vi "main.vi"() -> ()   [LabVIEW 2010]
uses:
  subVIs/XML_repo_library.lvlib
panel:
  out "MainLoop_state":T1(ring)
  in  "Tab Control":T2(tab)
  in  "Measure with":dbl(ring) items=["0. Demo Nanopositioner Stage 1.0", "0. Demo Avalanche Photodiode 1.0"]
  in  "Scan with":dbl(ring) items=["0. Demo Nanopositioner Stage 1.0", "0. Demo Avalanche Photodiode 1.0"]
  in  "stop":bool
  in  "start":bool
  in  "quit":bool
  out "Intensity Graph":dbl[][](graph)
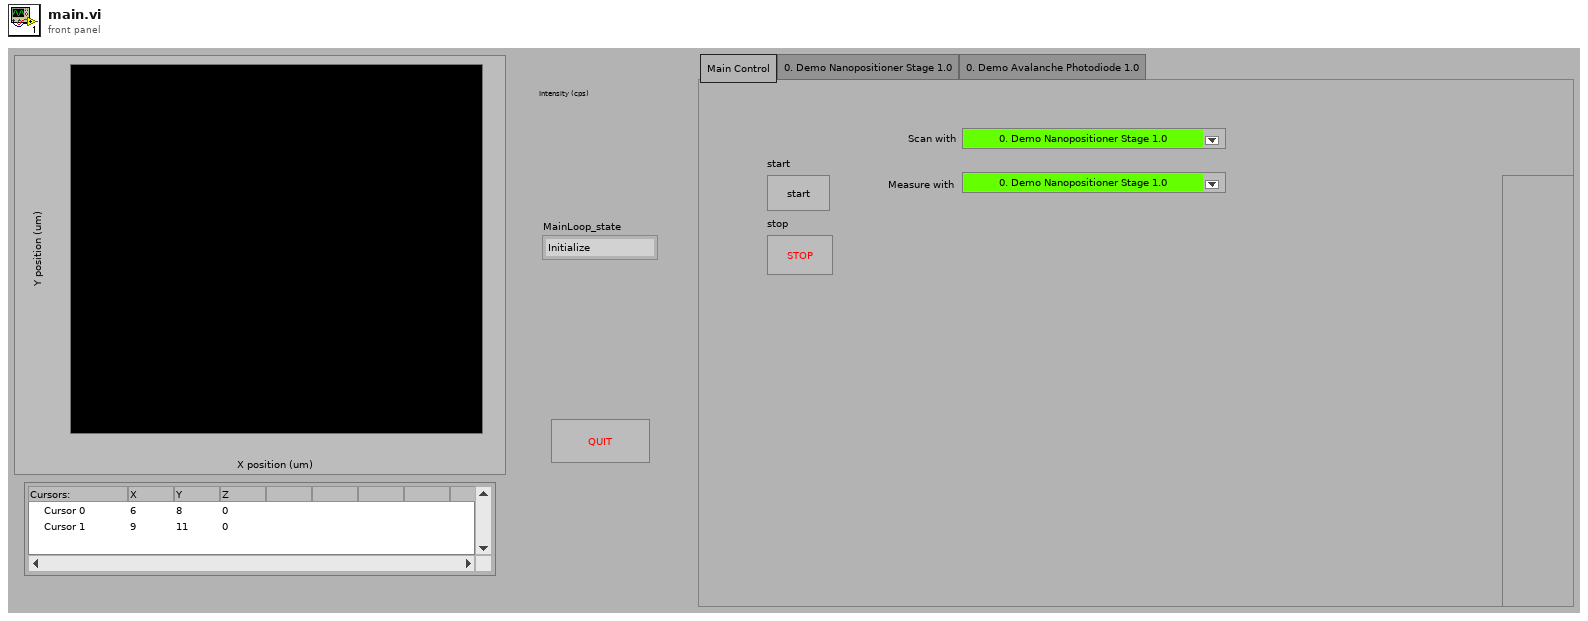
[diagram p1: front panel]
types:
  T1 = enum16{"Initialize", "Setup Elements", "IDLE", "Acquire", "Save to file", "Deinitialize", "Shutdown", ""}
  T2 = enum32{"Page 1", "Page 6", "Page 2", "Page 3", "Page 4", "Page 5", "Page 7", "Page 8"}
  T3 = cluster{"Name":string, "Setup_element_type":enum16{"positioner", "acquisition", "synchronized"}, "VIpath":path, "Return type":string, "Stage info":cluster{"Value":string, i32, "node text":string}[], "Number":u32, "Setup_element_direction":enum16{"output", "input", "io"}}[]
  T4 = cluster{"Name":string, "Setup_element_type":enum16{"positioner", "acquisition", "synchronized"}, "VIpath":path, "Return type":string, "Stage info":cluster{"Value":string, i32, "node text":string}[], "Number":u32, "Setup_element_direction":enum16{"output", "input", "io"}}
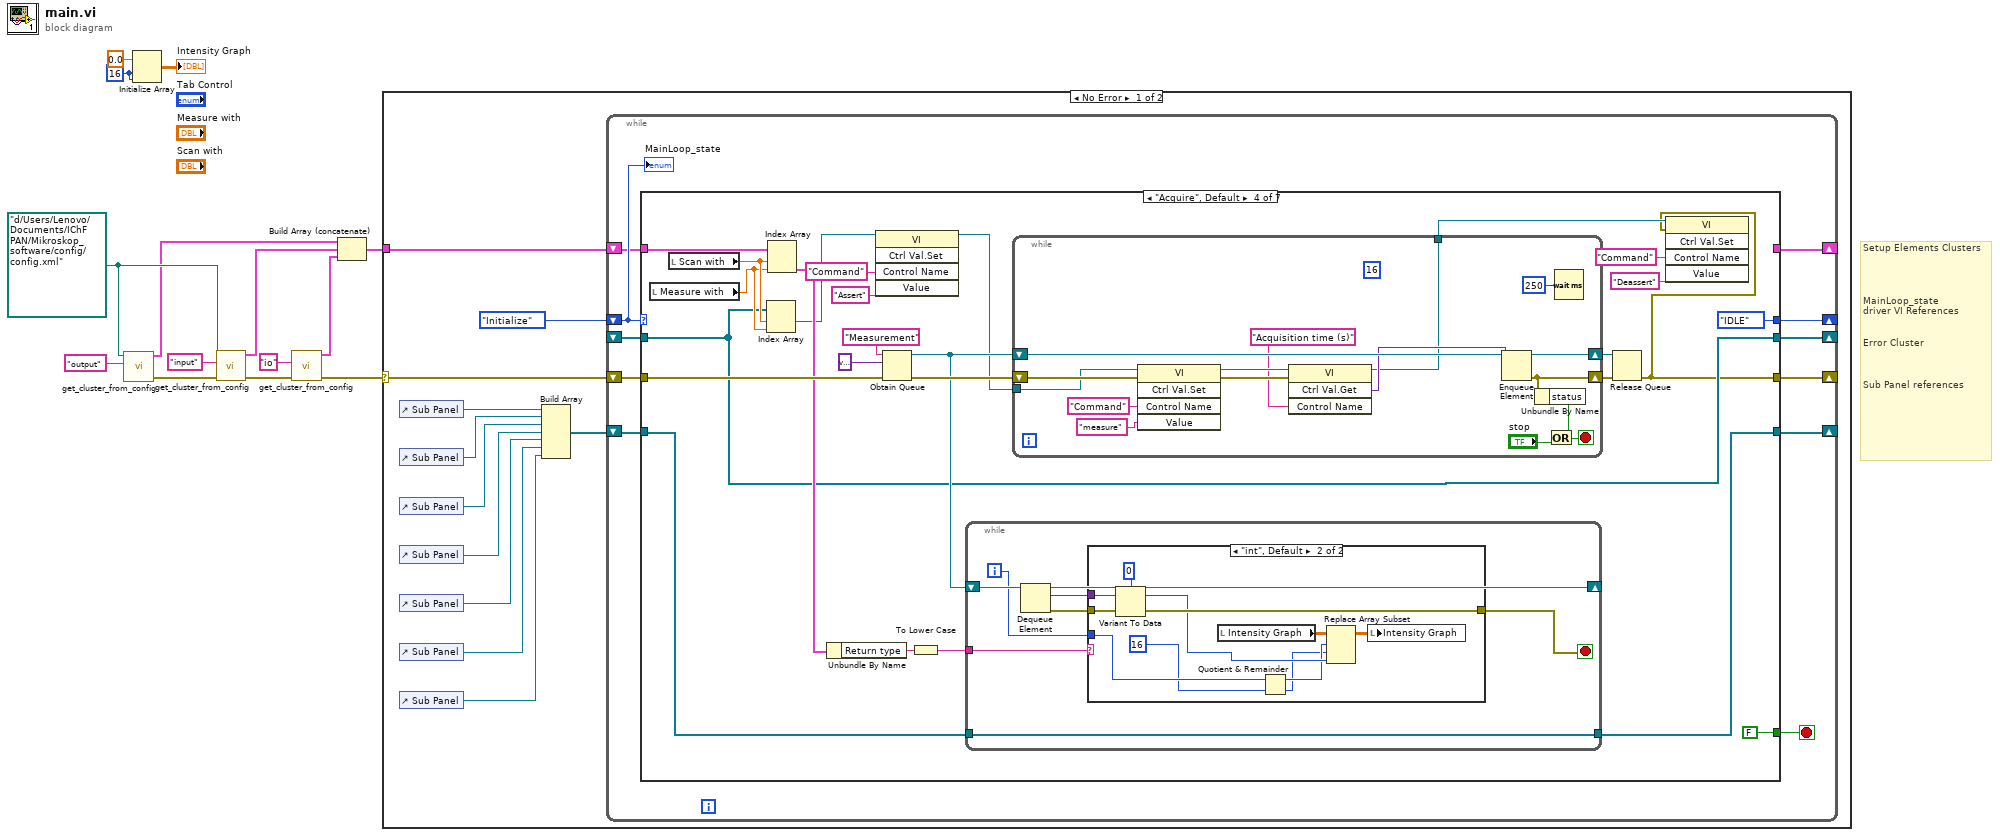
[diagram p0: block diagram]
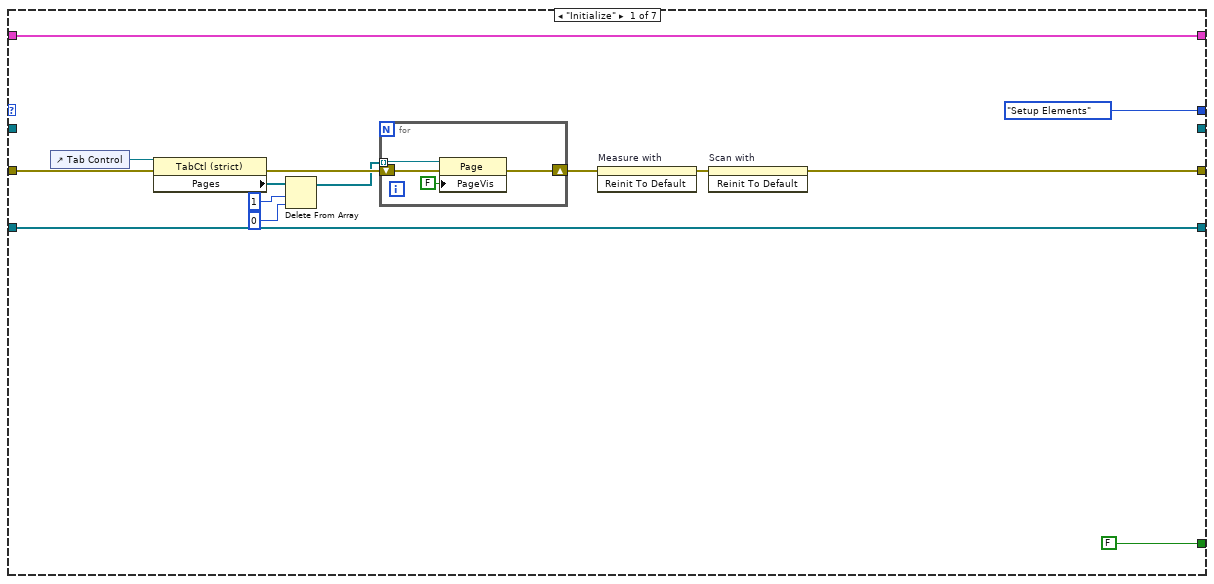
[diagram p2: hidden frame]
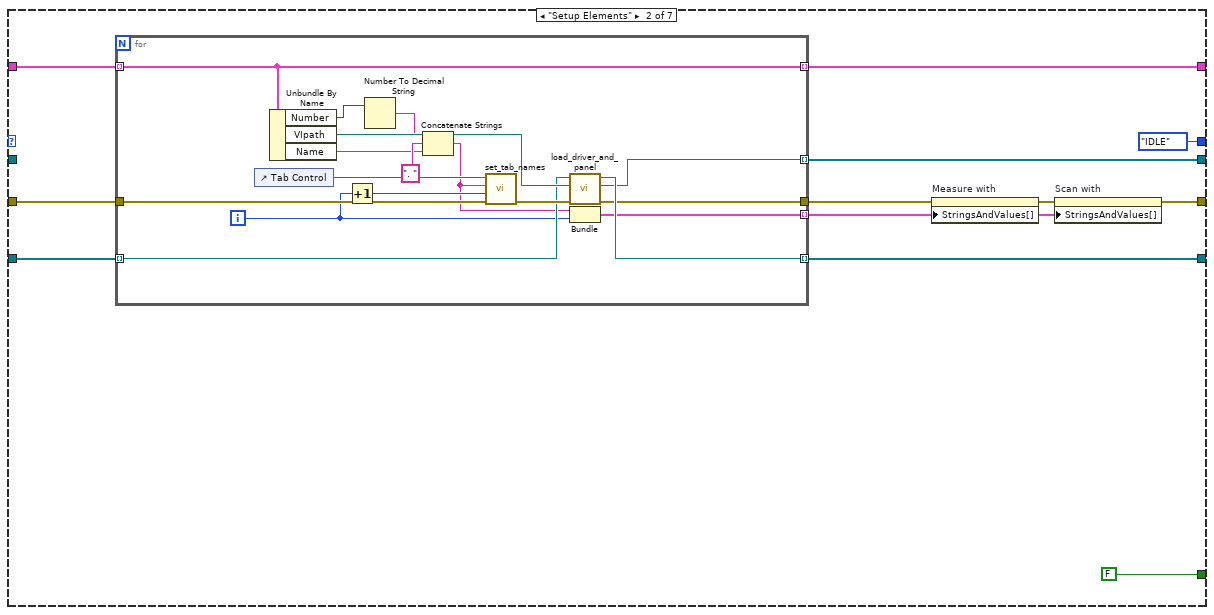
[diagram p3: hidden frame]
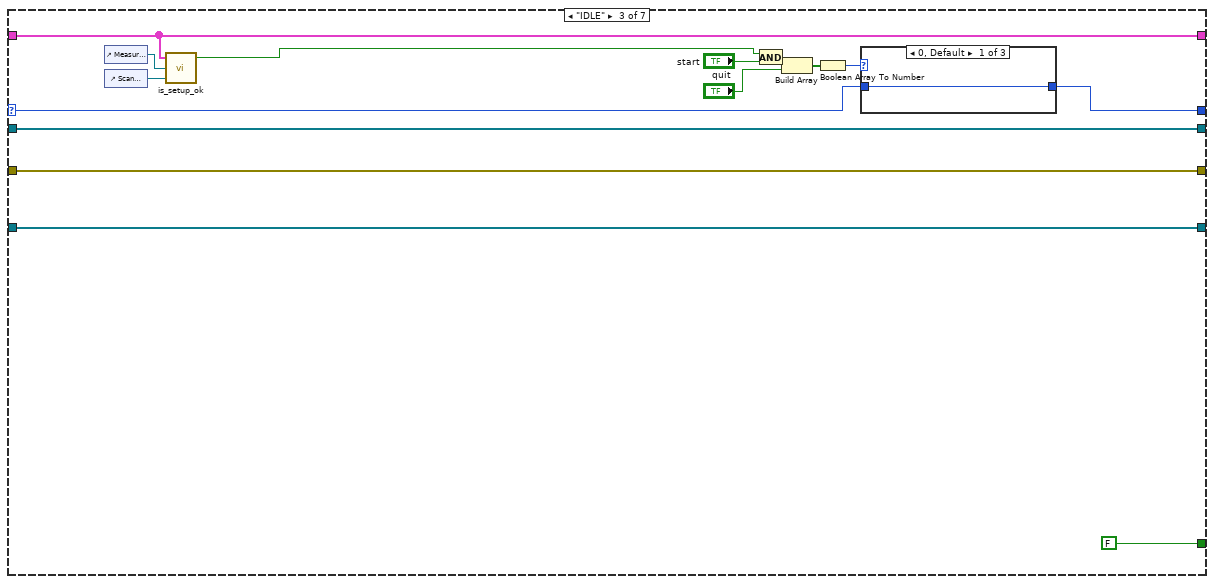
[diagram p4: hidden frame]
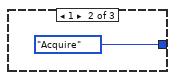
[diagram p5: hidden frame]
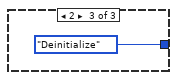
[diagram p6: hidden frame]
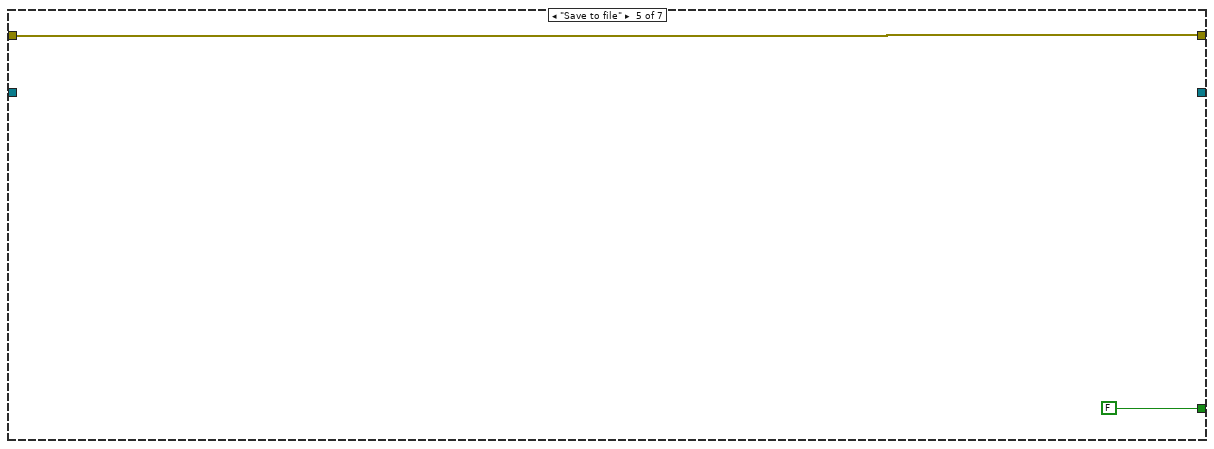
[diagram p8: hidden frame]
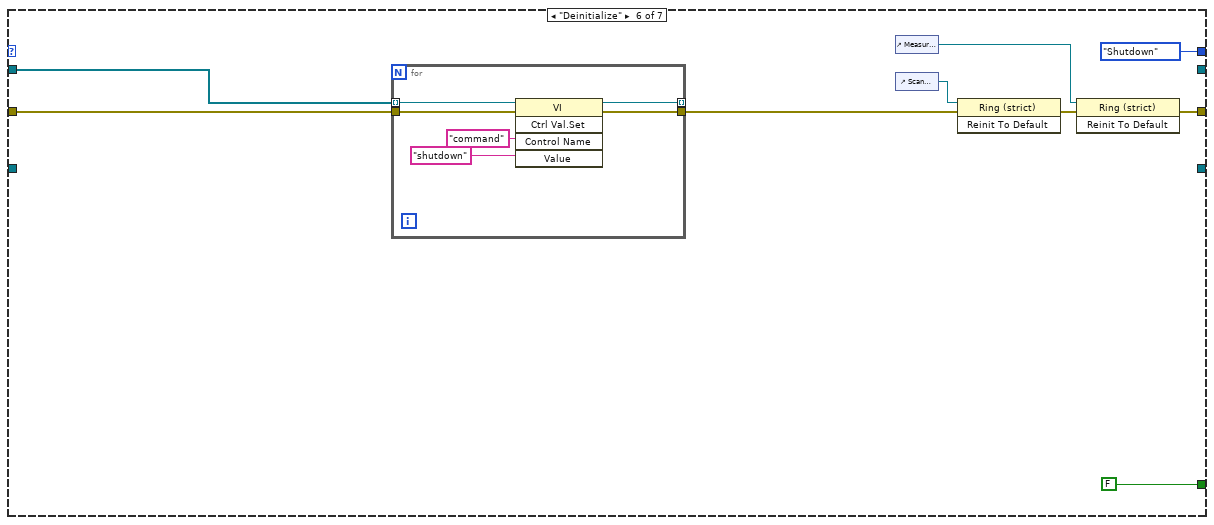
[diagram p9: hidden frame]
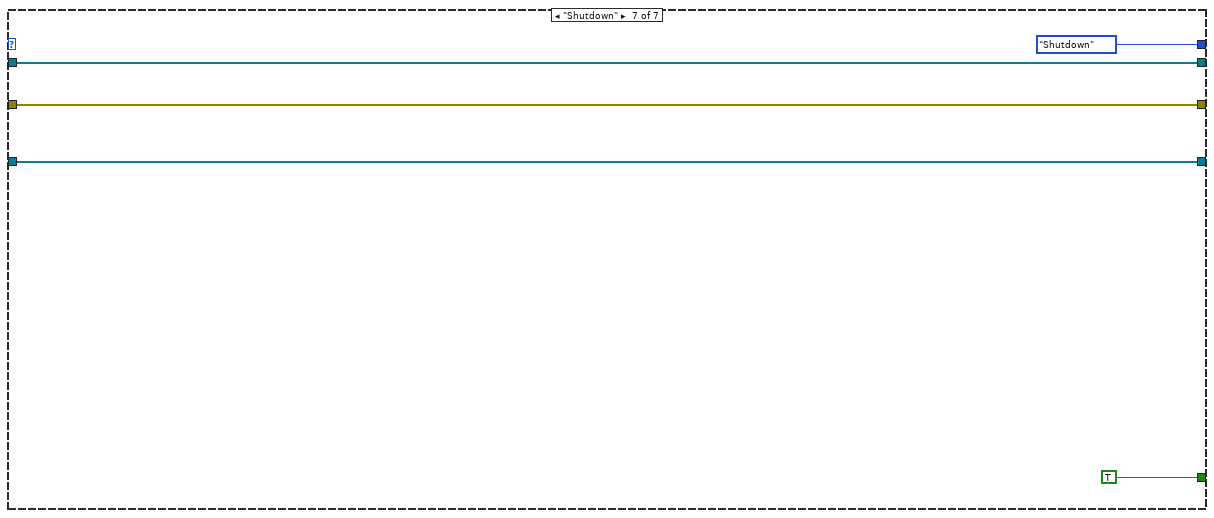
[diagram p10: hidden frame]
diagram:
  w1 = 16 ("dimension size")
  w12 = path "d:/Users/Lenovo/Documents/IChF PAN/Mikroskop_software/config/config.xml" ("path to XML document")
  # "Setup Elements Clusters\n\n\n\n\nMainLoop_state\ndriver VI References\n\n\nError Cluster\n\n\n\nSub Panel references"
  n1 = call "get_cluster_from_config.vi"("microscope tag type"="output" ("XPath expression"), "path to config file"=w12) -> ("error out"=w13:errorcluster, "Array"=w8:T3)  [unwired: 4 in]
  n2 = Initialize Array(0.0 ("element"), w1, w1) -> (→"Intensity Graph":dbl[][])
  n3 = call "get_cluster_from_config.vi"("error in (no error)"=w13, "microscope tag type"="input", "path to config file"=w12) -> ("error out"=w10:errorcluster, "Array"=w6:T3)  [unwired: 3 in]
  n4 = call "get_cluster_from_config.vi"("error in (no error)"=w10, "microscope tag type"="io") -> ("error out"=w4:errorcluster, "Array"=w5:T3)  [unwired: 4 in]
  n5 = Build Array (concatenate)(w8, w6, w5) -> (w7:T3)
  n6 = case shown="No Error" w4 {
    selector: w4 -> [w24 _]
    tunnel: w7 -> [w25 _]
    frame No Error {
      n7 = control-ref of="Sub Panel"() -> (w16:refnum<vi>)
      n8 = control-ref of="Sub Panel"() -> (w17:refnum<vi>)
      n9 = control-ref of="Sub Panel"() -> (w18:refnum<vi>)
      n10 = control-ref of="Sub Panel"() -> (w19:refnum<vi>)
      n11 = control-ref of="Sub Panel"() -> (w20:refnum<vi>)
      n12 = control-ref of="Sub Panel"() -> (w21:refnum<vi>)
      n13 = control-ref of="Sub Panel"() -> (w22:refnum<vi>)
      n14 = Build Array(w16, w17, w18, w19, w20, w21, w22) -> (w15:refnum<vi>[])
      n15 = while {
        shift-right: [w36] -> _
        shift-left: T1."Initialize" ("MainLoop_state") -> [w35]
        shift-right: [w33] -> _
        shift-left: w24 -> [w34]
        shift-right: [w30] -> _
        shift-left: w15 -> [w31]
        shift-right: [w29] -> _
        shift-left: w25 -> [w32]
        shift-right: [w27] -> _
        shift-left: _ -> [w26]
        stop <- w28 stop-if-true
        n16 = case shown="\"Acquire\", Default" w35 {
          selector: w35 -> [_ _ w89 _ _ _ _]
          tunnel: [T1."Setup Elements" ("MainLoop_state") T1."IDLE" ("MainLoop_state") w93 T1."IDLE" ("MainLoop_state") _ T1."Shutdown" ("MainLoop_state") T1."Shutdown" ("MainLoop_state")] -> w36
          tunnel: w34 -> [w44 w66 w90 w114 w165 w168 w182]
          tunnel: [w37 w55 w90 w102 w165 w171 w182] -> w33
          tunnel: w32 -> [w41 w62 w88 w116 _ _ _]
          tunnel: w31 -> [w42 w64 w98 w122 _ _ w181]
          tunnel: [w42 w63 w98 w123 _ _ w181] -> w30
          tunnel: [w41 w59 w88 _ _ _ _] -> w29
          tunnel: [FALSE FALSE FALSE FALSE FALSE FALSE TRUE] -> w28
          tunnel: [_ w60 w91 w110 _ _ w183] -> w27
          tunnel: w26 -> [_ _ w91 w110 _ w166 w183]
          frame "Initialize" {
            n17 = control-ref of="Tab Control"() -> (w50:refnum<vi>)
            n18 = property class="TabCtl (strict)"(reference=w50, error in=w44) -> (error out=w49:errorcluster, "Pages"=w48:refnum<vi>[])  [unwired: 1 out]
            n19 = Delete From Array(array=w48, length=1, index=0) -> (array with subset deleted=w47:refnum<vi>[])  [unwired: 1 out]
            n20 = for {
              tunnel: w47 -> [w53] mode=indexing
              shift-right: [w51] -> w38
              shift-left: w49 -> [w52]
              n21 = property class="Page"(reference=w53, error in=w52, "PageVis"=FALSE ("Page Visible")) -> (error out=w51:errorcluster)  [unwired: 1 out]
            }
            n22 = invoke on="Measure with" class="Ring (strict)" method="Reinit To Default"(error in=w38) -> (error out=w39:errorcluster)  [unwired: 2 in, 2 out]
            n23 = invoke on="Scan with" class="Ring (strict)" method="Reinit To Default"(error in=w39) -> (error out=w37:errorcluster)  [unwired: 2 in, 2 out]
          }
          frame "Setup Elements" {
            n24 = for {
              tunnel: w66 -> [w83]
              tunnel: [w67] -> w58
              tunnel: w62 -> [w72] mode=indexing
              tunnel: w64 -> [w77] mode=indexing
              tunnel: [w78] -> w63 mode=indexing
              tunnel: [w76] -> w60 mode=indexing
              tunnel: [w72] -> w59 mode=indexing
              tunnel: [w71] -> w56 mode=indexing
              i -> [w69]
              n25 = control-ref of="Tab Control"() -> (w82:refnum<vi>)
              n26 = Unbundle By Name(w72) -> ("Number"=w68:u32, "VIpath"=w79:path, "Name"=w73:string)
              n27 = Increment(x=w69) -> (x+1=w80:i32)
              n28 = Number To Decimal String(number=w68) -> (decimal integer string=w74:string)  [unwired: 1 in]
              n29 = Concatenate Strings(w74, ". " ("string"), w73) -> (w70:string)
              n30 = call "set_tab_names.vi"("error out 2"=w83, "index"=w80, "Name"=w70, "Tab Control"=w82) -> ("error out"=w81:errorcluster)  [unwired: 3 in]
              n31 = call "load_driver_and_panel.vi"("error in (no error)"=w81, "VIpath"=w79, "Sub Panel in"=w77) -> ("error out"=w67:errorcluster, "driver VI Refnum"=w76:refnum<vi>, "Sub Panel out"=w78:refnum<vi>)  [unwired: 2 in]
              n32 = Bundle(w70, w69) -> (w71:cluster{string, i32})  [unwired: 1 in]
            }
            n33 = property on="Measure with" class="Ring (strict)"(error in=w58, "StringsAndValues[]"=w56) -> (error out=w57:errorcluster)  [unwired: 1 in, 1 out]
            n34 = property on="Scan with" class="Ring (strict)"(error in=w57, "StringsAndValues[]"=w56) -> (error out=w55:errorcluster)  [unwired: 1 in, 1 out]
          }
          frame "IDLE" {
            n35 = control-ref of="Measure with"() -> (w86:refnum<vi>)
            n36 = control-ref of="Scan with"() -> (w85:refnum<vi>)
            n37 = call "is_setup_ok.vi"("Scan with"=w85, "Measure with"=w86, "Array"=w88) -> ("All OK"=w84:bool)  [unwired: 2 out]
            n38 = And(x=w84, y="start") -> (x .and. y?=w87:bool)
            n39 = Build Array(w87, "quit") -> (w95:bool[])
            n40 = Boolean Array To Number(Boolean array=w95) -> (number=w94:u32)
            n41 = case shown="0, Default" w94 {
              tunnel: [w99 T1."Acquire" ("MainLoop_state") T1."Deinitialize" ("MainLoop_state")] -> w93
              tunnel: w89 -> [w99 _ _]
              frame 0, Default {
              }
              frame 1 {
              }
              frame 2 {
              }
            }
          }
          frame "Acquire", Default {
            n42 = local read "Measure with"() -> (w111:dbl)
            n43 = local read "Scan with"() -> (w112:dbl)
            n44 = Index Array(array=w110, index #1=w112, index #2=w111) -> (element #1=w109:refnum<vi>)  [unwired: 1 out]
            n45 = Index Array(array=w116, index #1=w112, index #2=w111) -> (element #2=w113:T4)  [unwired: 1 out]
            n46 = Unbundle By Name(w113) -> ("Return type"=w115:string)
            n47 = invoke class="VI" method="Ctrl Val.Set"(reference=w109, "Control Name"="Command", "Value"="Assert" ("Control Name")) -> (reference out=w106:refnum<vi>)  [unwired: 2 in, 4 out]
            n48 = Obtain Queue(name (unnamed)="Measurement", element data type=variant ("variant"), error in (no error)=w114) -> (queue out=w126:refnum<queue>, error out=w127:errorcluster)  [unwired: 2 in, 1 out]
            n49 = To Lower Case(string=w115) -> (all lower case string=w117:string)
            n50 = while {
              shift-right: [w134] -> _
              shift-left: w126 -> [w135]
              tunnel: [w133] -> w123
              tunnel: w122 -> [w133]
              tunnel: w117 -> [w132]
              i -> [w128]
              stop <- w129 stop-if-true
              n51 = Dequeue Element(queue=w135) -> (queue out=w134:refnum<queue>, element=w131:variant, error out=w130:errorcluster)  [unwired: 2 in, 1 out]
              n52 = case shown="\"int\", Default" w132 {
                tunnel: w131 -> [_ w146]
                tunnel: w130 -> [w136 w145]
                tunnel: [w136 w144] -> w129
                tunnel: w128 -> [_ w140]
                frame "False" {
                }
                frame "int", Default {
                  n53 = Variant To Data(error in=w145, Variant=w146, type=0) -> (error out=w144:errorcluster, data=w141:i32)
                  n54 = local read "Intensity Graph"() -> (w142:dbl[][])
                  n55 = Quotient & Remainder(x=w140, y=16) -> (x-y*floor(x/y)=w138:i32, floor(x/y)=w137:i32)
                  n56 = Replace Array Subset(array=w142, new element=w141, index (row)=w138, index (col)=w137) -> (w143:dbl[][])
                  n57 = local write "Intensity Graph"(w143) -> ()
                }
              }
            }
            n58 = while {
              shift-right: [w162] -> w124
              shift-left: w127 -> [w156]
              shift-right: [w158] -> w125
              shift-left: w126 -> [w163]
              tunnel: w106 -> [w154]
              tunnel: [w148] -> w103
              stop <- w160 stop-if-true
              (unwired) 16 ("dimension size")
              n59 = invoke class="VI" method="Ctrl Val.Set"(reference=w154, error in=w156, "Control Name"="Command", "Value"="measure" ("Control Name")) -> (reference out=w151:refnum<vi>, error out=w152:errorcluster)  [unwired: 1 in, 3 out]
              n60 = invoke class="VI" method="Ctrl Val.Get"(reference=w151, error in=w152, "Control Name"="Acquisition time (s)") -> (reference out=w148:refnum<vi>, "Get Control Value Variant"=w149:variant)  [unwired: 1 in, 2 out]
              n61 = Enqueue Element(queue=w163, element=w149) -> (queue out=w158:refnum<queue>, error out=w162:errorcluster)  [unwired: 2 in, 1 out]
              n62 = Unbundle By Name(w162) -> ("status"=w161:bool)
              n63 = Or(x=w161, y="stop") -> (x .or. y?=w160:bool)
              n64 = Wait (ms)(milliseconds to wait=u32 250) -> ()  [unwired: 1 out]
            }
            n65 = Release Queue(queue=w125, error in (no error)=w124) -> (error out=w102:errorcluster)  [unwired: 1 in, 2 out]
            n66 = invoke class="VI" method="Ctrl Val.Set"(reference=w103, error in=w102, "Control Name"="Command", "Value"="Deassert" ("Control Name")) -> ()  [unwired: 1 in, 5 out]
          }
          frame "Save to file" {
          }
          frame "Deinitialize" {
            n67 = for {
              tunnel: w168 -> [w178]
              tunnel: [w177] -> w167
              tunnel: [w176] -> _ mode=indexing
              tunnel: w166 -> [w175] mode=indexing
              n68 = invoke class="VI" method="Ctrl Val.Set"(reference=w175, error in=w178, "Control Name"="command", "Value"="shutdown" ("Control Name")) -> (reference out=w176:refnum<vi>, error out=w177:errorcluster)  [unwired: 1 in, 3 out]
            }
            n69 = control-ref of="Measure with"() -> (w169:refnum<vi>)
            n70 = control-ref of="Scan with"() -> (w170:refnum<vi>)
            n71 = invoke on="Invoke Node" class="Ring (strict)" method="Reinit To Default"(reference=w170, error in=w167) -> (error out=w172:errorcluster)  [unwired: 1 in, 2 out]
            n72 = invoke on="Invoke Node" class="Ring (strict)" method="Reinit To Default"(reference=w169, error in=w172) -> (error out=w171:errorcluster)  [unwired: 1 in, 2 out]
          }
          frame "Shutdown" {
          }
        }
        "MainLoop_state" <- w35
      }
    }
    frame Error {
    }
  }
